vi "InbetweenDist1point.vi"(7 "Inbetween diff":dbl=3.0, 8 "Z":dbl, 9 "X":dbl, 10 "Index":i32, 11 "All Lines":T1) -> (0 "Bad   In angle?":bool, 1 "Lower index":i32, 2 "In range?":bool)   [LabVIEW 2014]
uses:
  Libraries/Map Data Folder/All-Lines.ctl
  Libraries/Map Data Folder/LineCluster.ctl
  Libraries/Map Data Folder/LineConnection.ctl
  Libraries/Map Data Folder/Map Data.lvlib
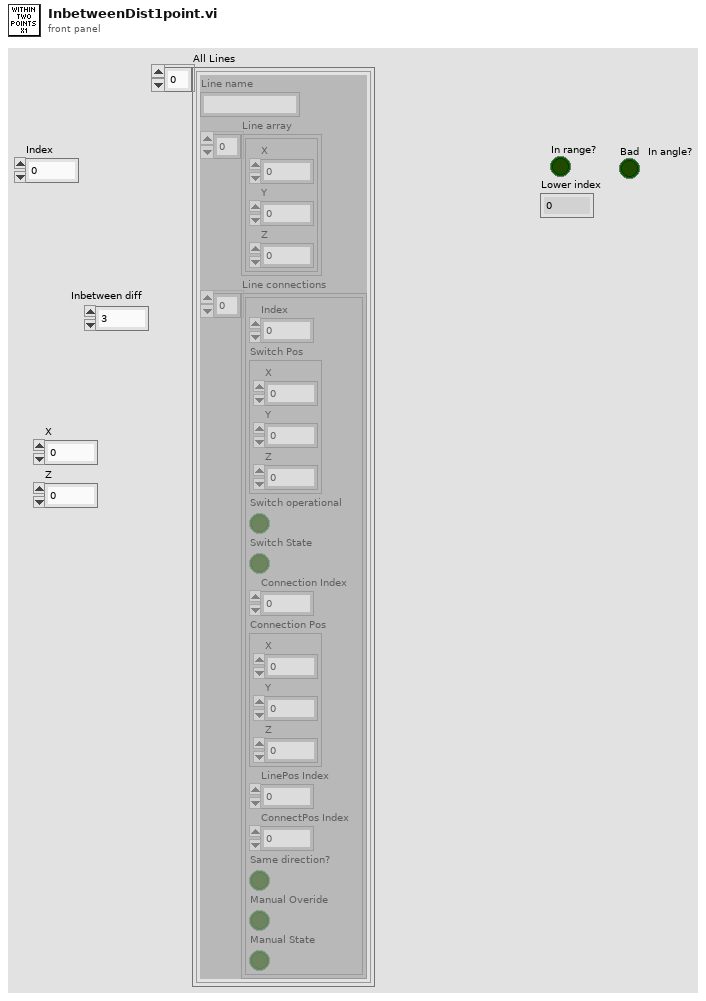
[diagram p1: front panel]
types:
  T1 = typedef "Map Data.lvlib/All-Lines.ctl" = T2[]
  T2 = typedef "Map Data.lvlib/LineCluster.ctl" = cluster{"Line name":string, "Line array":cluster{"X":dbl, "Y":dbl, "Z":dbl}[], "Line connections":T3[]}
  T3 = typedef "LineConnection.ctl" = cluster{"Index":i32, "Switch Pos":cluster{"X":dbl, "Y":dbl, "Z":dbl}, "Switch operational":bool, "Switch State":bool, "Connection Index":i32, "Connection Pos":cluster{"X":dbl, "Y":dbl, "Z":dbl}, "LinePos Index":i32, "ConnectPos Index":i32, "Same direction?":bool, "Manual Overide":bool, "Manual State":bool}
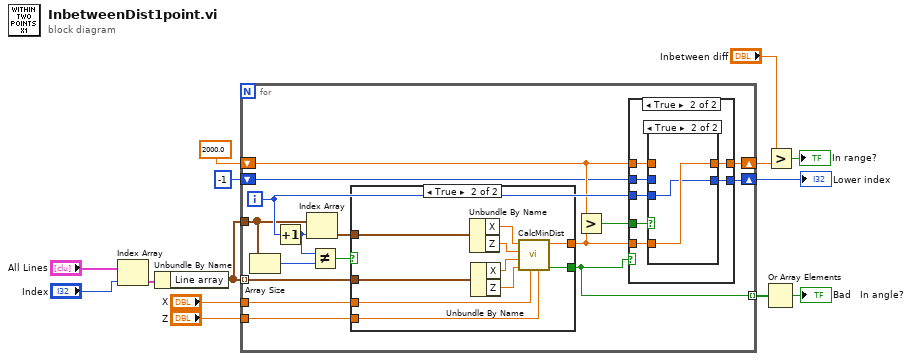
[diagram p0: block diagram]
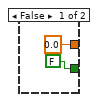
[diagram p2: hidden frame]
diagram:
  n1 = Index Array(array="All Lines", index="Index") -> (element=w14:T2)
  n2 = Unbundle By Name(w14) -> ("Line array"=w11:cluster{"X":dbl, "Y":dbl, "Z":dbl}[])
  n3 = for {
    tunnel: w11 -> [w30] mode=indexing
    tunnel: w11 -> [w21]
    shift-right: [w27] -> w9
    shift-left: 2000.0 ("Result") -> [w26]
    shift-right: [w24] -> w5
    shift-left: -1 -> [w23]
    tunnel: [w18] -> w4 mode=indexing
    tunnel: "X" -> [w16]
    tunnel: "Z" -> [w15]
    i -> [w29]
    n4 = Array Size(array=w21) -> (size(s)=w17:i32)
    n5 = Increment(x=w29) -> (x+1=w19:i32)
    n6 = Index Array(array=w21, index=w19) -> (element=w22:cluster{"X":dbl, "Y":dbl, "Z":dbl})
    n7 = Not Equal?(x=w19, y=w17) -> (x != y?=w20:bool)
    n8 = case shown="True" w20 {
      tunnel: w30 -> [_ w39]
      tunnel: [0.0 ("Result") w42] -> w28
      tunnel: w22 -> [_ w40]
      tunnel: [FALSE ("Inbetween?") w41] -> w18
      tunnel: w16 -> [_ w34]
      tunnel: w15 -> [_ w33]
      frame False {
      }
      frame True {
        n9 = Unbundle By Name(w40) -> ("X"=w36:dbl, "Z"=w35:dbl)
        n10 = Unbundle By Name(w39) -> ("X"=w38:dbl, "Z"=w37:dbl)
        n11 = call "CalcMinDist.vi"("PointY"=w33, "PointX"=w34, "Line2Y"=w37, "Line2X"=w38, "Line1Y"=w35, "Line1X"=w36) -> ("In Angle?"=w41:bool, "Result"=w42:dbl)  [unwired: 4 in]
      }
    }
    n12 = Greater?(x=w26, y=w28) -> (0:w25:bool)
    n13 = case shown="True" w18 {
      tunnel: w28 -> [_ w50]
      tunnel: w29 -> [_ w46]
      tunnel: w26 -> [w44 w48]
      tunnel: [w44 w49] -> w27
      tunnel: w25 -> [_ w51]
      tunnel: [w43 w47] -> w24
      tunnel: w23 -> [w43 w45]
      frame False {
      }
      frame True {
        n14 = case shown="True" w51 {
          tunnel: w50 -> [_ w55]
          tunnel: [w53 w55] -> w49
          tunnel: w48 -> [w53 _]
          tunnel: [w52 w54] -> w47
          tunnel: w46 -> [_ w54]
          tunnel: w45 -> [w52 _]
          frame False {
          }
          frame True {
          }
        }
      }
    }
  }
  "Lower index" <- w5
  n15 = Or Array Elements(Boolean array=w4) -> (logical OR=→"Bad   In angle?":bool)
  n16 = Greater?(x="Inbetween diff", y=w9) -> (0:→"In range?":bool)
